vi "IsoPlane_Device.vi"(7 "Device-specific in":variant, 8 "error in (no error)":errorcluster, 10 "Position in":dbl[](array[numeric]), 11 "Operation":T2(ring)) -> (0 "error out":errorcluster, 1 "Device properties":cluster{"Axes":string[], "Tolerance":dbl[][]}, 2 "Position out":dbl[](array[numeric]), 3 "Status":T1, 5 "Device-specific out":variant)   [LabVIEW 2018]
uses:
  ProgramData/Documents/Princeton Instruments/LightField/Add-in and Automation SDK/Samples/LabVIEW Automation/lightfield-automation-labview/LightField Automation.lvclass
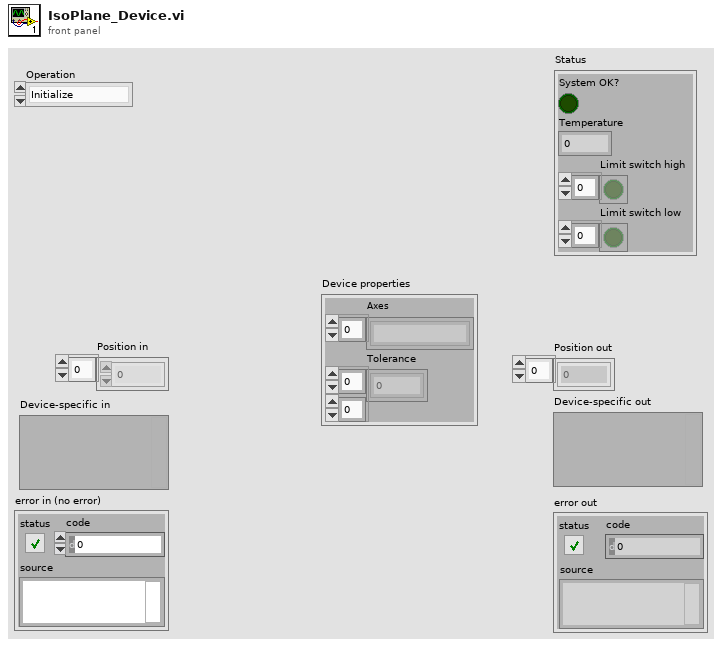
[diagram p1: front panel]
types:
  T1 = cluster{"System OK?":bool, "Temperature":dbl, "Limit switch high":bool[], "Limit switch low":bool[]}
  T2 = enum16{"Initialize", "Shut down", "Set position", "Get position", "Get status", "Other settings"}
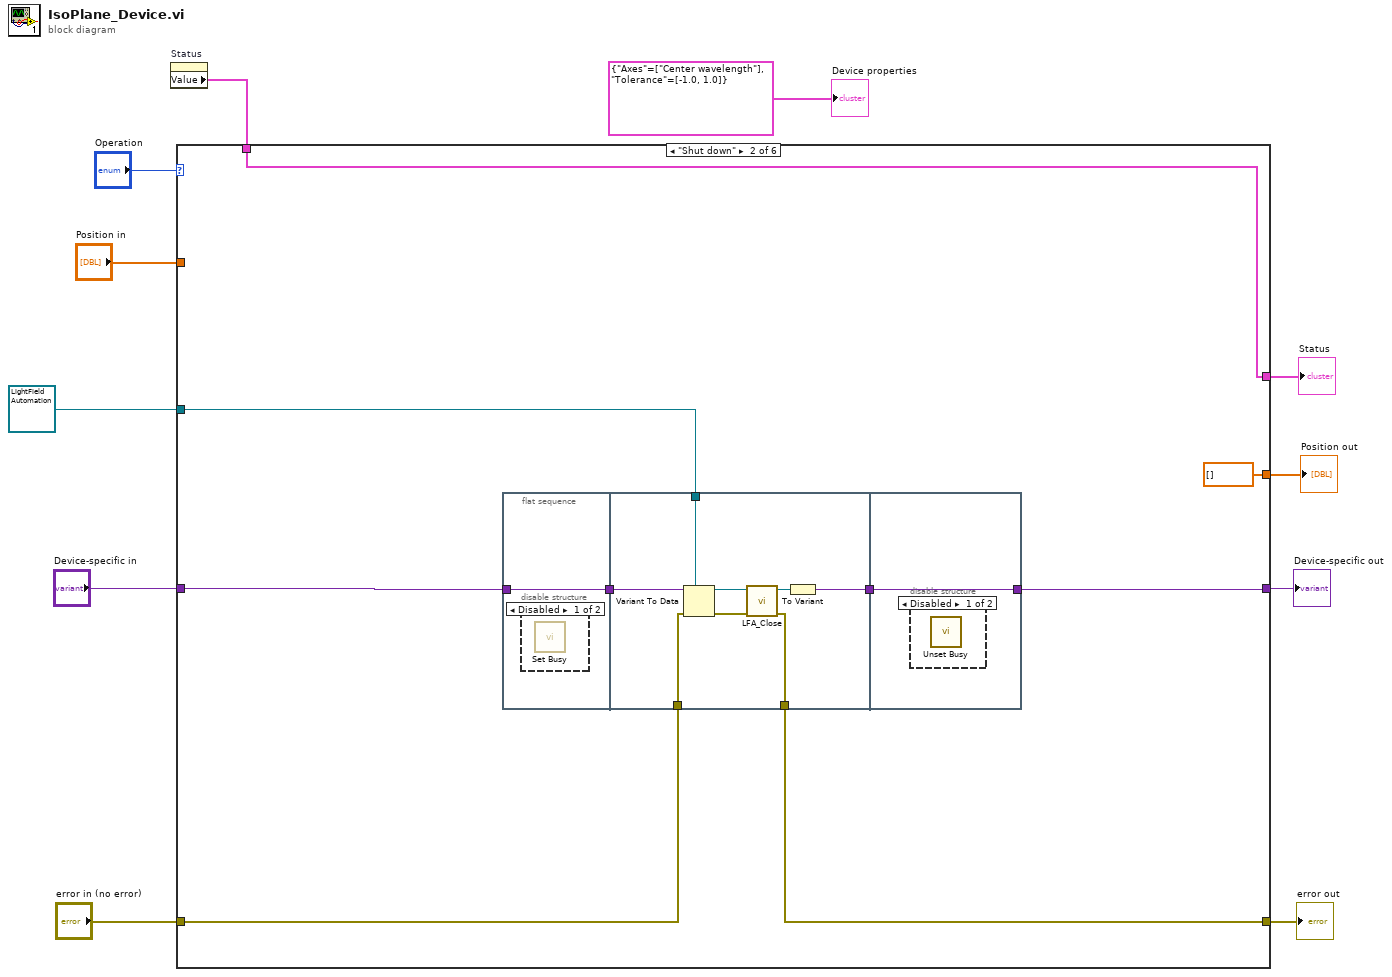
[diagram p0: block diagram]
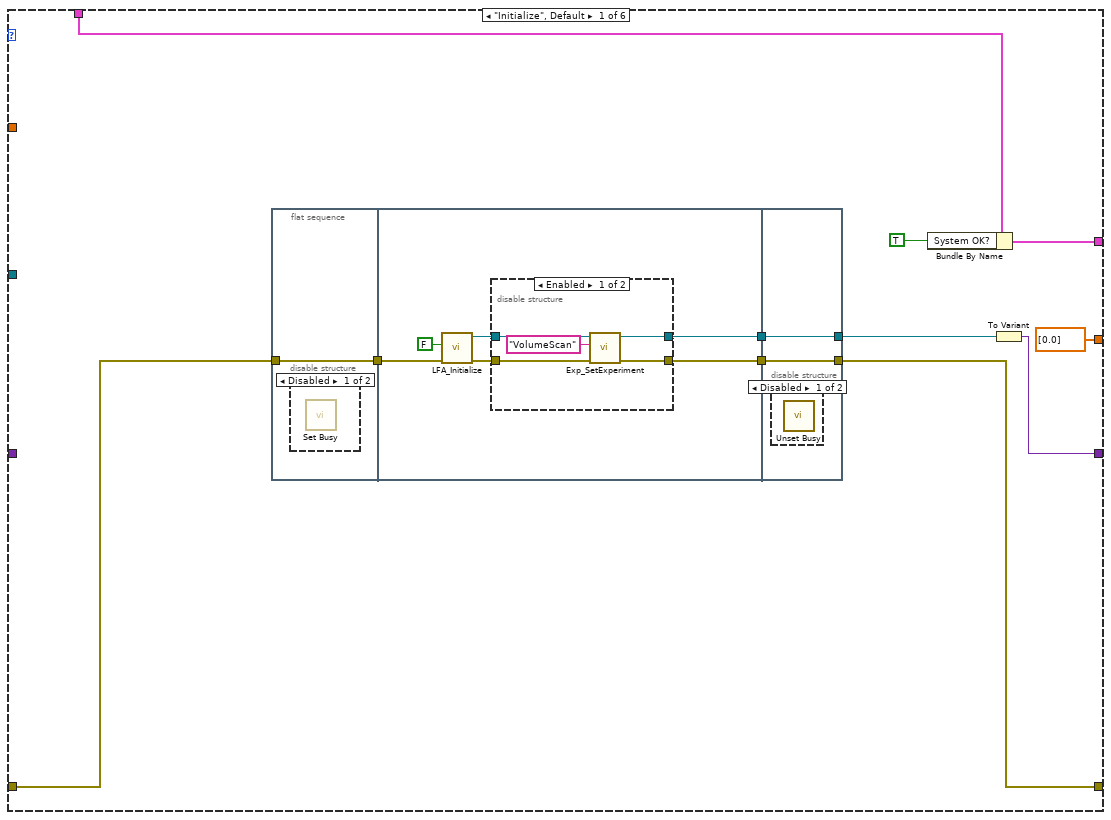
[diagram p2: hidden frame]
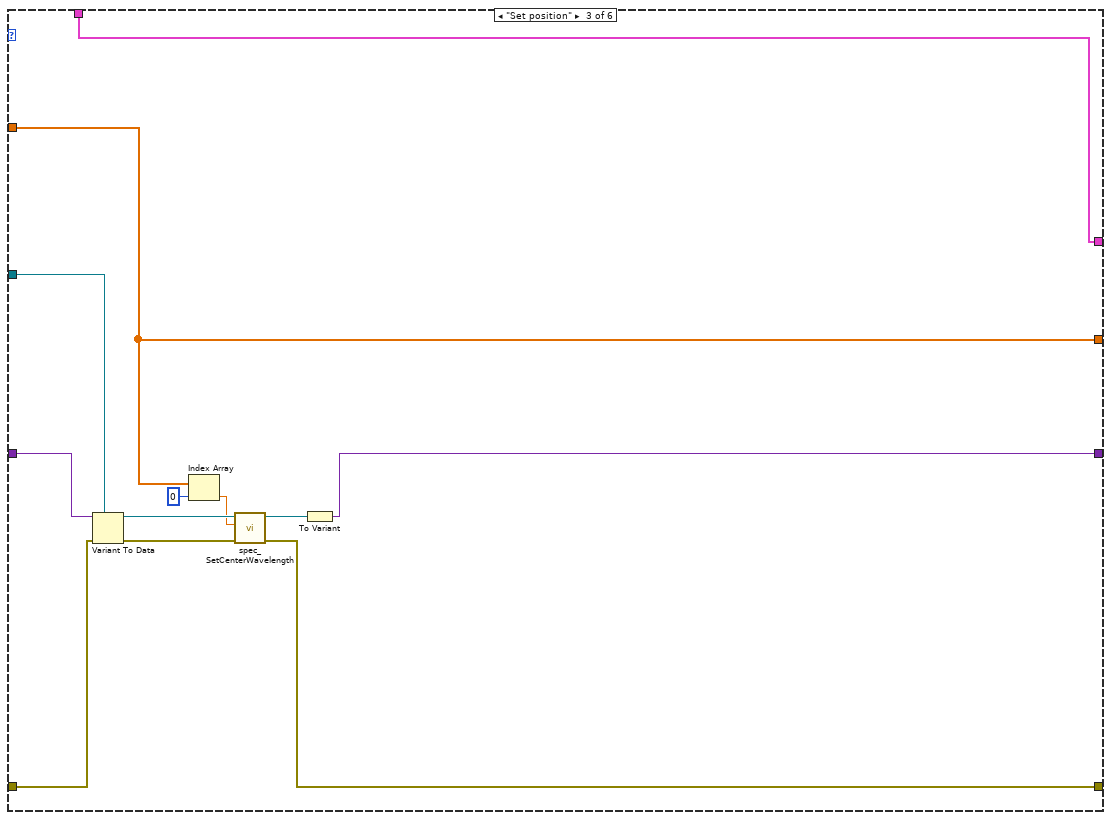
[diagram p8: hidden frame]
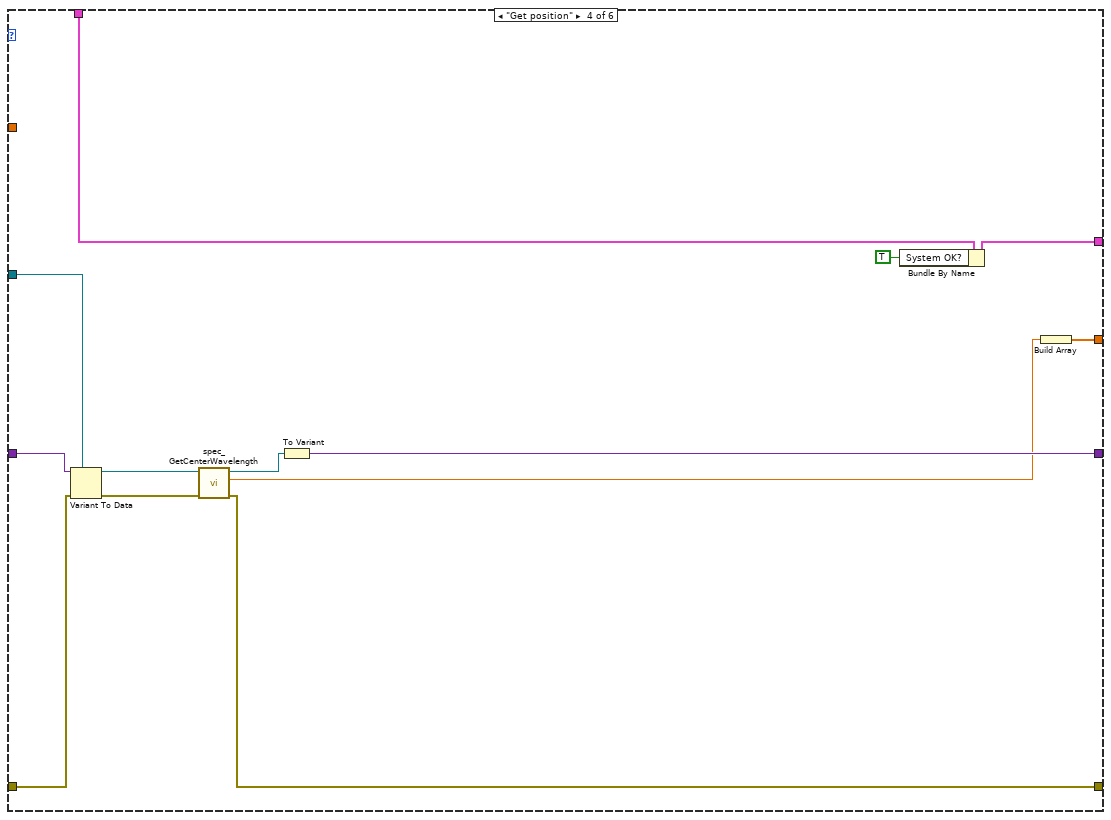
[diagram p9: hidden frame]
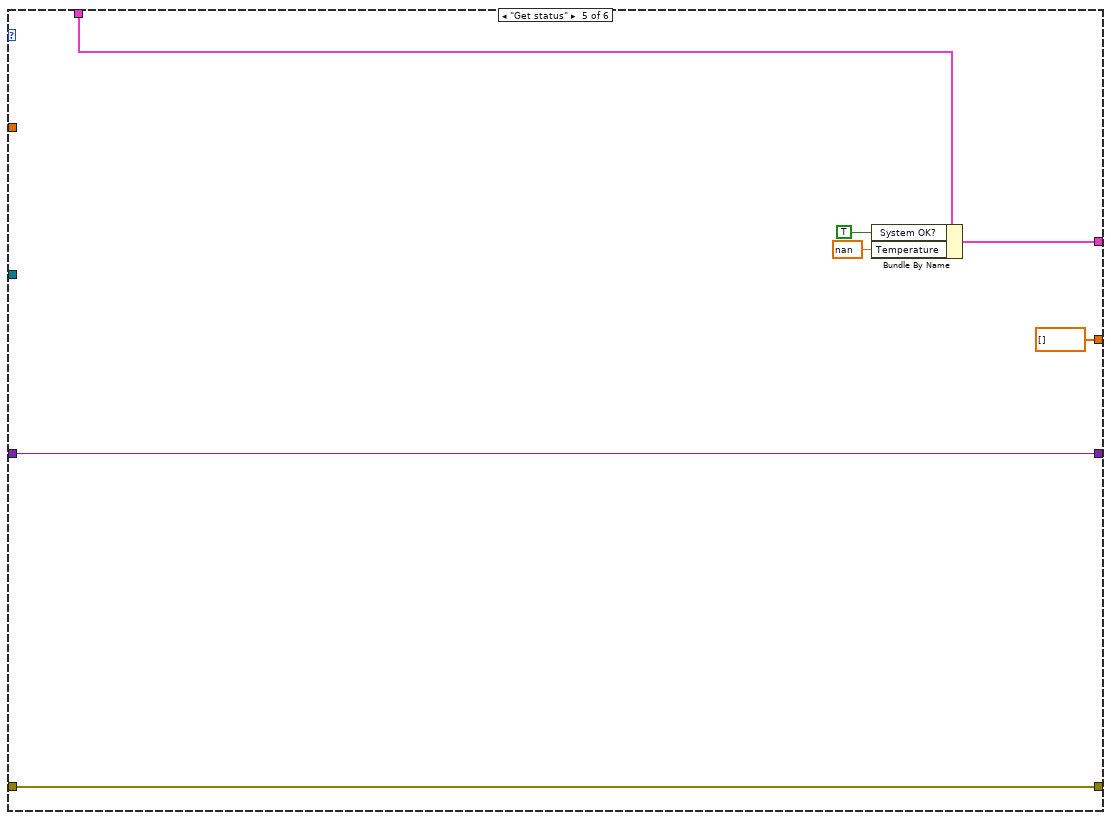
[diagram p10: hidden frame]
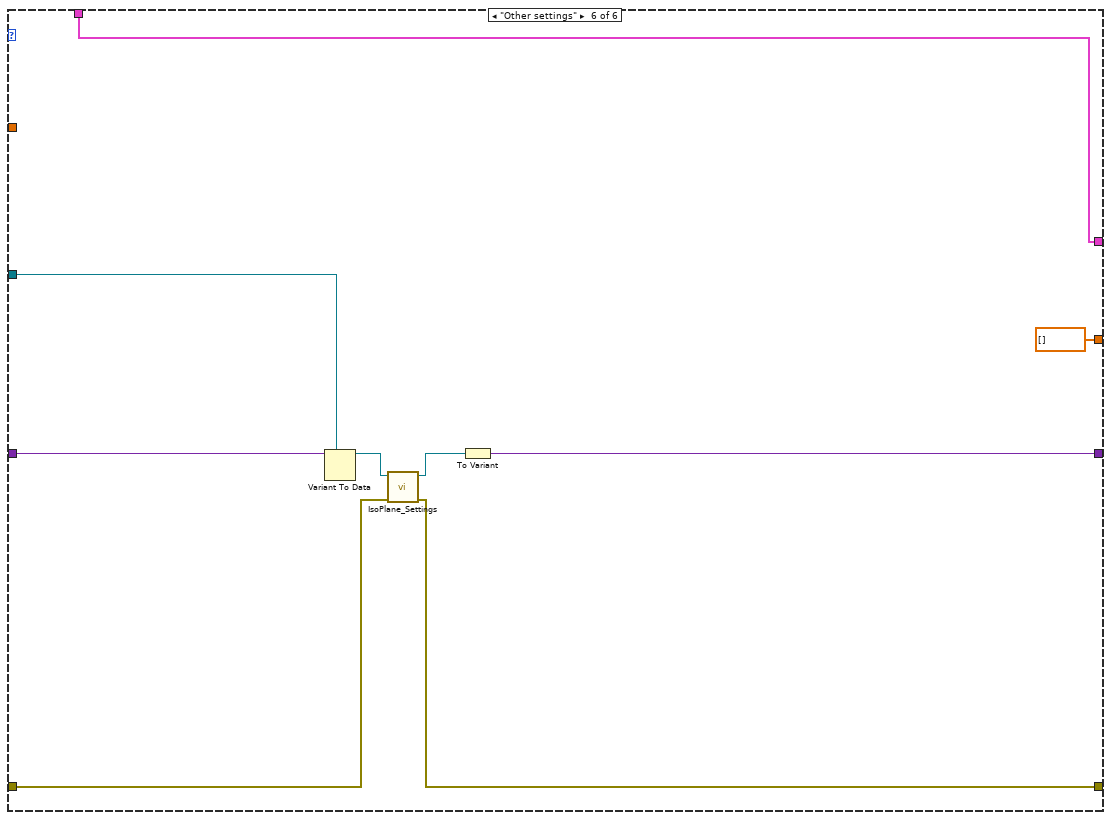
[diagram p11: hidden frame]
diagram:
  n1 = property on="Status" class="Clust (strict)"() -> ("Value"=w10:T1)  [unwired: 2 in, 2 out]
  n2 = case shown="\"Shut down\"" "Operation" {
    tunnel: "Position in" -> [_ _ w66 _ _ _]
    tunnel: w10 -> [w22 w47 w69 w82 w89 w98]
    tunnel: [w21 w47 w69 w81 w88 w98] -> w9
    tunnel: "Device-specific in" -> [_ w44 w62 w79 w85 w96]
    tunnel: [dbl[] [0.0] ("Position in") dbl[] [] ("Position in") w66 w73 dbl[] [] ("Position in") dbl[] [] ("Position in")] -> w6
    tunnel: [w18 w43 w61 w77 w85 w92] -> w5
    tunnel: [w15 w41 w58 w70 w84 w90] -> w4
    tunnel: "error in (no error)" -> [w17 w42 w59 w71 w84 w91]
    tunnel: refnum<class "LightField Automation.lvclass"> refnum ("LightField Automation out") -> [_ w45 w68 w78 _ w95]
    frame "Initialize", Default {
      n3 = flat-sequence {
        tunnel: w17 -> [w23]
        tunnel: [w23] -> w12
        tunnel: [w25] -> w14
        tunnel: [w24] -> w13
        tunnel: w12 -> [w27]
        tunnel: [w37] -> w15
        tunnel: [w38] -> w16
        tunnel: w14 -> [w38]
        tunnel: w13 -> [w37]
        frame #0 {
          n4 = disable-structure shown="Disabled" {
            frame Disabled {
              n5 = call <vilib>:"Set Busy.vi"() -> ()  [unwired: 10 in, 2 out]
            }
            frame Enabled {
            }
          }
        }
        frame #1 {
          n6 = call "LFA_Initialize.vi"("error in (no error)"=w27, "Is Visible?"=FALSE) -> ("error out"=w28:errorcluster, "LightField Automation out"=w29:refnum<class "LightField Automation.lvclass">)  [unwired: 8 in]
          n7 = disable-structure shown="Enabled" {
            disable-tunnel: w29 -> [w34 w36]
            disable-tunnel: [w32 w36] -> w25
            disable-tunnel: w28 -> [w31 w35]
            disable-tunnel: [w30 w35] -> w24
            frame Enabled {
              n8 = call "Exp_SetExperiment.vi"("error in (no error)"=w31, "ExperimentName"="VolumeScan", "LightField Automation in"=w34) -> ("error out"=w30:errorcluster, "LightField Automation out"=w32:refnum<class "LightField Automation.lvclass">)  [unwired: 7 in]
            }
            frame Disabled {
            }
          }
        }
        frame #2 {
          n9 = disable-structure shown="Disabled" {
            frame Disabled {
              n10 = call <vilib>:"Unset Busy.vi"() -> ()  [unwired: 11 in, 1 out]
            }
            frame Enabled {
            }
          }
        }
      }
      n11 = Bundle By Name(cluster=w22, "System OK?"=TRUE) -> (w21:T1)
      n12 = To Variant(anything=w16) -> (Variant=w18:variant)
    }
    frame "Shut down" {
      n13 = flat-sequence {
        tunnel: w44 -> [w48]
        tunnel: [w48] -> w40
        tunnel: w45 -> [w56]
        tunnel: w42 -> [w50]
        tunnel: [w49] -> w41
        tunnel: w40 -> [w55]
        tunnel: [w52] -> w39
        tunnel: [w57] -> w43
        tunnel: w39 -> [w57]
        frame #0 {
          n14 = disable-structure shown="Disabled" {
            frame Disabled {
              n15 = call <vilib>:"Set Busy.vi"() -> ()  [unwired: 10 in, 2 out]
            }
            frame Enabled {
            }
          }
        }
        frame #1 {
          n16 = Variant To Data(error in=w50, type=w56, Variant=w55) -> (data=w54:refnum<class "LightField Automation.lvclass">, error out=w51:errorcluster)
          n17 = call "LFA_Close.vi"("error in (no error)"=w51, "LightField Automation in"=w54) -> ("error out"=w49:errorcluster, "LightField Automation out"=w53:refnum<class "LightField Automation.lvclass">)  [unwired: 8 in]
          n18 = To Variant(anything=w53) -> (Variant=w52:variant)
        }
        frame #2 {
          n19 = disable-structure shown="Disabled" {
            frame Disabled {
              n20 = call <vilib>:"Unset Busy.vi"() -> ()  [unwired: 11 in, 1 out]
            }
            frame Enabled {
            }
          }
        }
      }
    }
    frame "Set position" {
      n21 = Variant To Data(error in=w59, type=w68, Variant=w62) -> (data=w67:refnum<class "LightField Automation.lvclass">, error out=w64:errorcluster)
      n22 = Index Array(array=w66, index=0) -> (element=w65:dbl)
      n23 = call "spec_SetCenterWavelength.vi"("error in (no error)"=w64, "Center Wavelength"=w65, "LightField Automation in"=w67) -> ("error out"=w58:errorcluster, "LightField Automation out"=w63:refnum<class "LightField Automation.lvclass">)  [unwired: 7 in]
      n24 = To Variant(anything=w63) -> (Variant=w61:variant)
    }
    frame "Get position" {
      n25 = Variant To Data(error in=w71, type=w78, Variant=w79) -> (data=w76:refnum<class "LightField Automation.lvclass">, error out=w72:errorcluster)
      n26 = call "spec_GetCenterWavelength.vi"("error in (no error)"=w72, "LightField Automation in"=w76) -> ("error out"=w70:errorcluster, "Center Wavelenght"=w74:dbl, "LightField Automation out"=w75:refnum<class "LightField Automation.lvclass">)  [unwired: 7 in]
      n27 = To Variant(anything=w75) -> (Variant=w77:variant)
      n28 = Bundle By Name(cluster=w82, "System OK?"=TRUE) -> (w81:T1)
      n29 = Build Array(w74) -> (w73:dbl[])
    }
    frame "Get status" {
      n30 = Bundle By Name(cluster=w89, "System OK?"=TRUE, "Temperature"=nan) -> (w88:T1)
    }
    frame "Other settings" {
      n31 = Variant To Data(type=w95, Variant=w96) -> (data=w94:refnum<class "LightField Automation.lvclass">)  [unwired: 1 in, 1 out]
      n32 = call "IsoPlane_Settings.vi"("error in (no error)"=w91, "LightField Automation in"=w94) -> ("error out"=w90:errorcluster, "LightField Automation out"=w93:refnum<class "LightField Automation.lvclass">)  [unwired: 8 in]
      n33 = To Variant(anything=w93) -> (Variant=w92:variant)
    }
  }
  "Status" <- w9
  "Device-specific out" <- w5
  "error out" <- w4
  "Position out" <- w6
  "Device properties" <- cluster{"Axes":string[], "Tolerance":dbl[][]} {"Axes"=["Center wavelength"], "Tolerance"=[[-1.0, 1.0]]} ("Device properties")
